vi "STATUS_Main.vi"() -> (11 "ConfigFile":path=path "/home/ArcVIEW/Modules/TCSP60/config/TCSP60_Default.cfg")   [LabVIEW 2016]
doc: "Main VI for the COMSTCP Module. This module is in charge of the externl TCP/IP comunications"
uses:
  DBSHAND/private/vis/DatabaseHand_Element_Set(string).vi
  DBSHAND/private/vis/DatabaseHand_Element_Get(string).vi
panel:
  in  "enabled":bool
  in  "updateprog":bool
  out "stop":bool
  in  "cmdstruct":cluster{"cmd":string, "respQ":string}
  out "last async.":string
  out "async":refnum<k5>
  out "error out 2":errorcluster
  in  "maxrate":sgl=0.5
  in  "maxasyncinst":i8=2
  in  "Log":bool
  in  "logfile":path
  in  "serverport":u16
  out "error out":errorcluster
  in  "Initialization Variables":string[][](table)=[["Comms", "serverport", "STATUS_Main.vi", "serverport", "1501", "U16"], ["Comms", "maxinst", "STATUS_Main.vi", "maxinst", "", "U8"], ["Misc", "maxrate", "STATUS_Main.vi", "maxrate", "", "FLOAT"], ["Misc", "updateprog", "STATUS_Main.vi", "updateprog", "", "BOOL"], ["Misc", "enabled", "STATUS_Main.vi", "enabled", "", "BOOL"], ["LOG", "file", "STATUS_Main.vi", "logfile", "", "PATH"], ["LOG", "log", "STATUS_Main.vi", "Log", "", "BOOL"]]
  in  "error in":errorcluster
  in  "ModuleName":string="STATUS"
  out "stopped":bool=TRUE
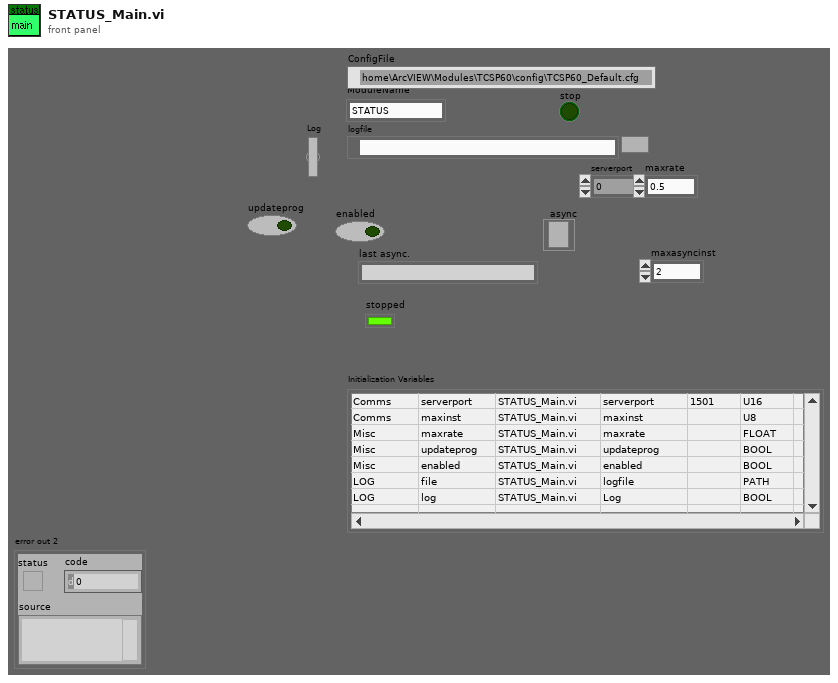
[diagram p1: front panel]
types:
  T1 = enum16{"get", "send", "delete", "add", "clean", "send_all", "send_on", "send_off"}
  T2 = typedef "DatabaseHand_RefNum.ctl" = refnum<vi>
  T3 = typedef "Status_VarsStruct.ctl" = cluster{"name":string, "value":string, "last":u32, "max":u32}
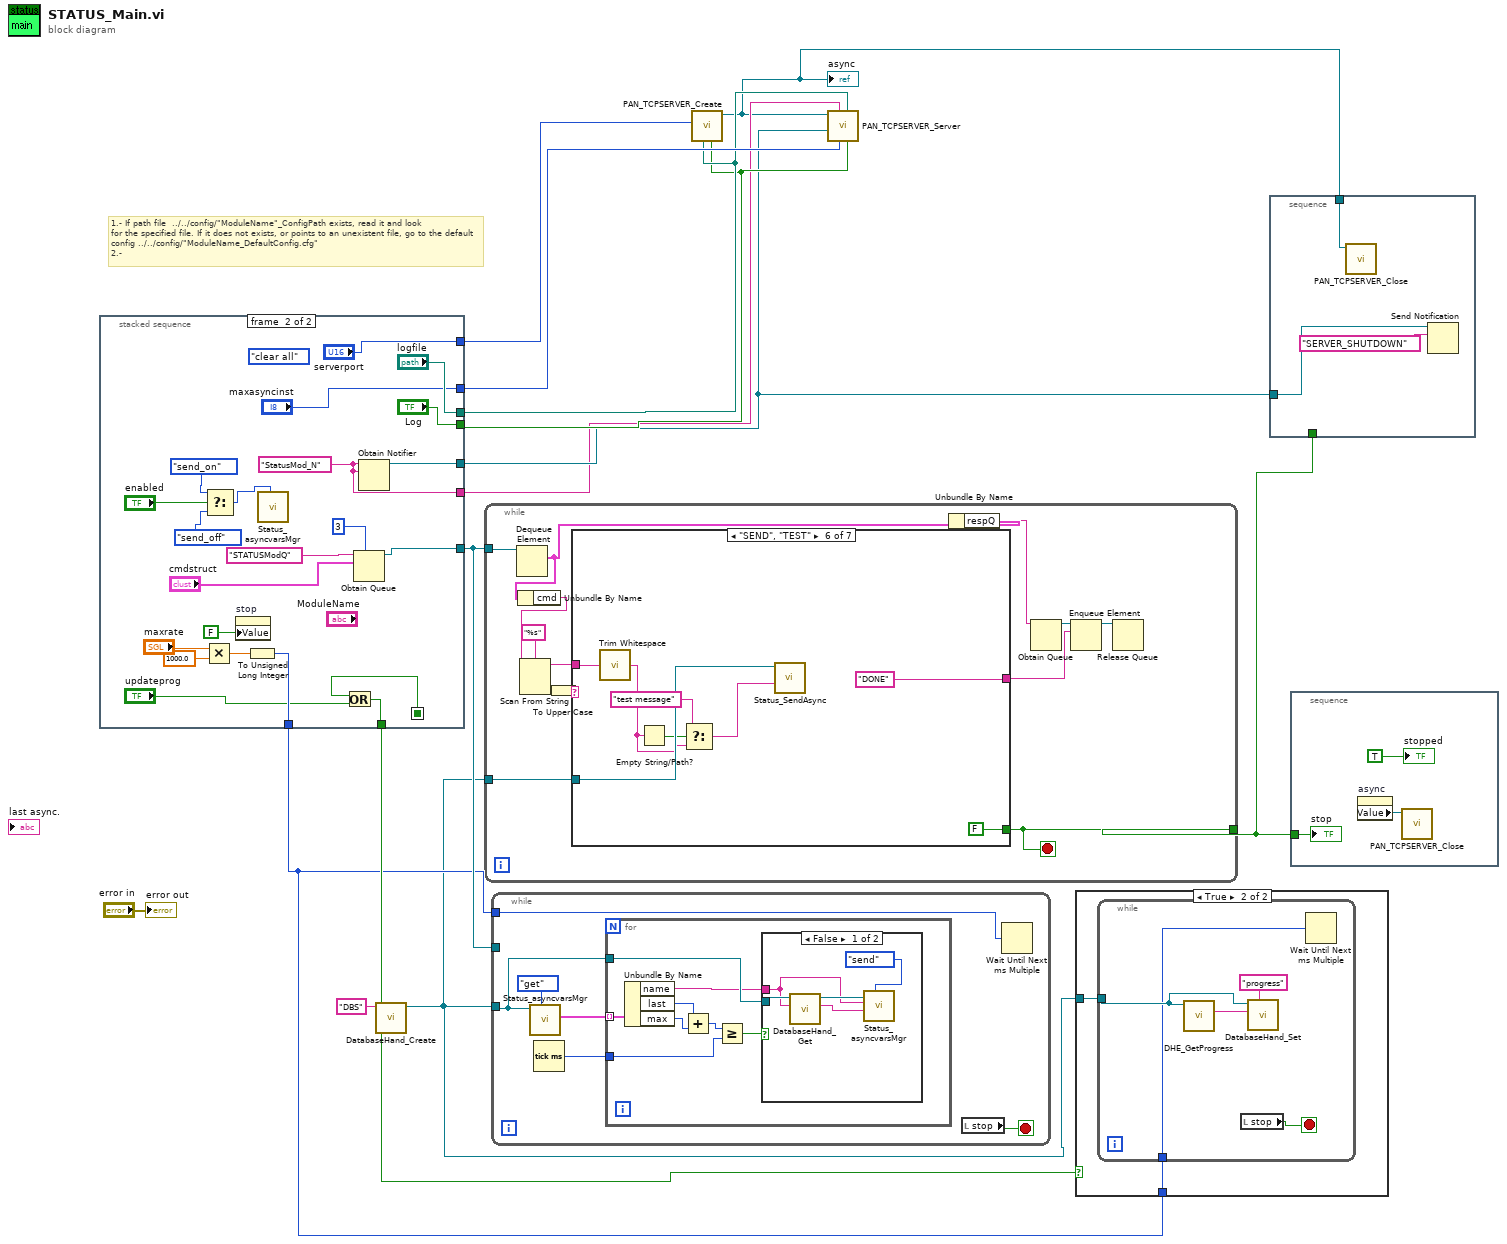
[diagram p0: block diagram]
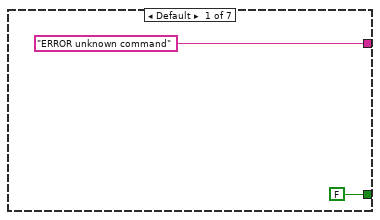
[diagram p4: hidden frame]
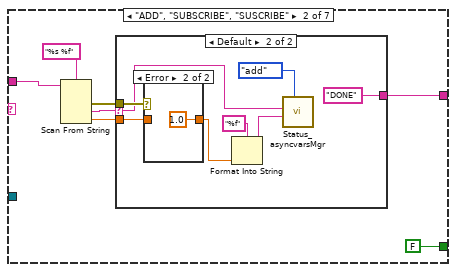
[diagram p5: hidden frame]
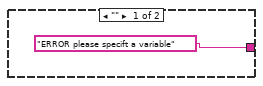
[diagram p6: hidden frame]
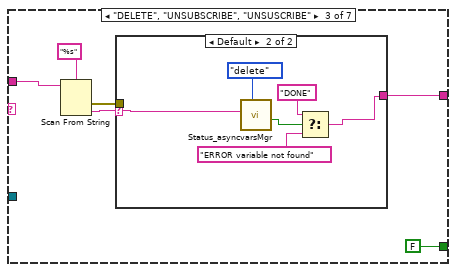
[diagram p8: hidden frame]
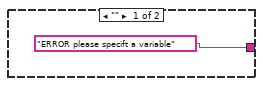
[diagram p9: hidden frame]
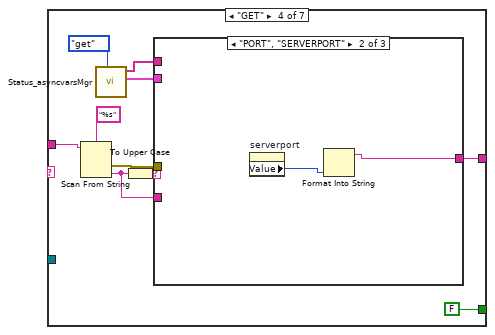
[diagram p10: hidden frame]
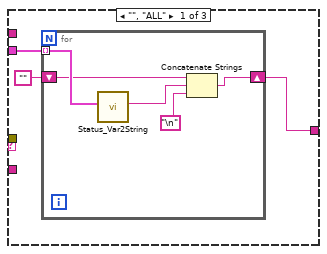
[diagram p11: hidden frame]
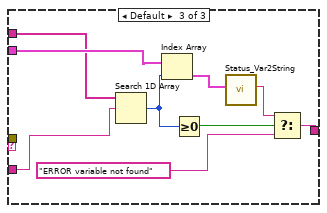
[diagram p12: hidden frame]
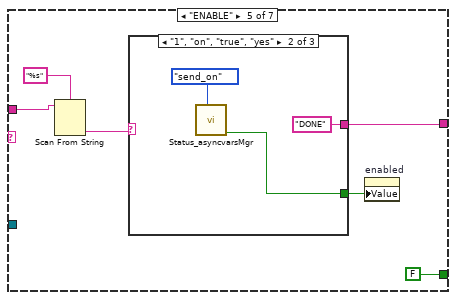
[diagram p13: hidden frame]
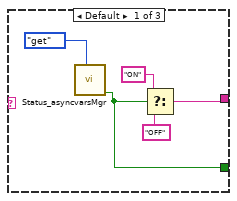
[diagram p14: hidden frame]
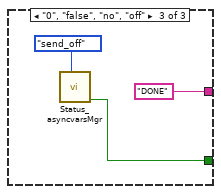
[diagram p15: hidden frame]
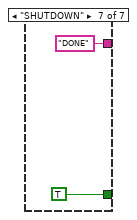
[diagram p16: hidden frame]
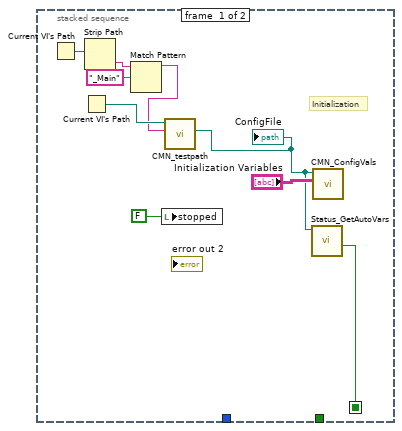
[diagram p17: hidden frame]
diagram:
  # "1.- If path file  ../../config/\"ModuleName\"_ConfigPath exists, read it and look\nfor the specified file. If it does not exists, or points to an unexistent file, go to the default\nconfig ../../config/\"ModuleName_DefaultConfig.cfg\"\n2.-"
  n1 = stacked-sequence {
    seq-local: [w15 _] -> [_ w25]
    tunnel: [_ "maxasyncinst"] -> w14
    tunnel: [_ "logfile"] -> w12
    tunnel: [_ "Log"] -> w11
    tunnel: [_ w43] -> w10
    tunnel: [_ w42] -> w9
    tunnel: [_ "serverport"] -> w8
    tunnel: [_ w36] -> w7
    tunnel: [_ w31] -> w2
    tunnel: [_ w24] -> w5
    frame #0 {
      # "Initialization"
      n2 = Current VI's Path() -> (path=w18:path)
      n3 = Current VI's Path() -> (path=w21:path)
      n4 = Strip Path(path=w18) -> (name=w19:string)  [unwired: 1 out]
      n5 = Match Pattern(string=w19, regular expression="_Main") -> (before substring=w17:string)  [unwired: 4 out]
      n6 = local write "stopped"(FALSE ("stopped")) -> ()
      n7 = call "CMN_testpath.vi"("ModuleName"=w17, "caller Path"=w21) -> ("ConfigFile"=w16:path)  [unwired: 1 in, 8 out]
      "ConfigFile" <- w16
      n8 = call "Status_GetAutoVars.vi"("ConfigFile"=w16) -> ("progress"=w15:bool)  [unwired: 1 in, 9 out]
      n9 = call "CMN_ConfigVals.vi"("ConfigVariables"="Initialization Variables", "configuration file path"=w16) -> ()  [unwired: 2 in, 8 out]
    }
    frame #1 {
      w42 = "StatusMod_N" ("name (unnamed)")
      (unwired) enum16{"add", "delete", "find", "clear all"}."clear all" ("action")
      n10 = Multiply(x="maxrate", y=sgl 1000.0) -> (x*y=w32:sgl)
      n11 = Select(t=T1."send_on" ("action"), s="enabled", f=T1."send_off" ("action")) -> (s? t:f=w28:T1)
      n12 = property on="stop" class="Bool (strict)"("Value"=FALSE ("stop")) -> ()  [unwired: 2 in, 2 out]
      n13 = To Unsigned Long Integer(number=w32) -> (unsigned 32bit integer=w31:u32)
      n14 = call "Status_asyncvarsMgr.vi"("action"=w28) -> ()  [unwired: 4 in, 7 out]
      n15 = Or(x=w25, y="updateprog") -> (x .or. y?=w24:bool)
      n16 = Obtain Queue(max queue size (-1, unlimited)=3, name (unnamed)="STATUSModQ", element data type="cmdstruct") -> (queue out=w36:refnum<queue>)  [unwired: 2 in, 2 out]
      n17 = Obtain Notifier(name (unnamed)=w42, notification data type=w42) -> (notifier out=w43:refnum<notifier>)  [unwired: 2 in, 2 out]
    }
  }
  n18 = call "DatabaseHand_Create.vi"("Name"="DBS") -> ("Database RefNum out"=w1:T2)  [unwired: 1 in, 9 out]
  n19 = while {
    tunnel: w7 -> [w58]
    tunnel: [w54] -> w3
    tunnel: w1 -> [w46]
    stop <- w54 stop-if-true
    n20 = Dequeue Element(queue=w58) -> (element=w53:cluster{"cmd":string, "respQ":string})  [unwired: 1 in, 4 out]
    n21 = Unbundle By Name(w53) -> ("cmd"=w57:string)
    n22 = Scan From String(format string="%s", input string=w57) -> (remaining string=w48:string, output 1=w55:string)  [unwired: 2 in, 3 out]
    n23 = To Upper Case(1:w55) -> (0:w47:string)
    n24 = case shown="\"SEND\", \"TEST\"" w47 {
      tunnel: [FALSE FALSE FALSE FALSE FALSE FALSE TRUE] -> w54
      tunnel: ["ERROR unknown command" ("element") w63 w80 w98 w122 "DONE" ("element") "DONE" ("element")] -> w49
      tunnel: w48 -> [_ w66 w83 w100 w125 w142 _]
      tunnel: w46 -> [_ _ _ _ _ w143 _]
      frame Default {
      }
      frame "ADD", "SUBSCRIBE", "SUSCRIBE" {
        n25 = Scan From String(format string="%s %f", input string=w66) -> (error out=w61:errorcluster, output 1=w64:string, output 2=w62:dbl)  [unwired: 2 in, 4 out]
        n26 = case shown="Default" w64 {
          selector: w64 -> [_ w73]
          tunnel: ["ERROR please specift a variable" ("element") "DONE" ("element")] -> w63
          tunnel: w62 -> [_ w75]
          tunnel: w61 -> [_ w76]
          frame "" {
          }
          frame Default {
            n27 = case shown="Error" w76 {
              tunnel: w75 -> [w77 _]
              tunnel: [w77 1.0] -> w72
              frame No Error {
              }
              frame Error {
              }
            }
            n28 = Format Into String(format string="%f", w72) -> (resulting string=w71:string)  [unwired: 2 in, 1 out]
            n29 = call "Status_asyncvarsMgr.vi"("action"=T1."add", "value"=w71, "var"=w73) -> ()  [unwired: 2 in, 7 out]
          }
        }
      }
      frame "DELETE", "UNSUBSCRIBE", "UNSUSCRIBE" {
        n30 = Scan From String(format string="%s", input string=w83) -> (error out=w79:errorcluster, output 1=w81:string)  [unwired: 2 in, 3 out]
        n31 = case shown="Default" w81 {
          selector: w81 -> [_ w90]
          tunnel: ["ERROR please specift a variable" ("element") w87] -> w80
          tunnel: w79 -> [_ _]
          frame "" {
          }
          frame Default {
            n32 = call "Status_asyncvarsMgr.vi"("action"=T1."delete", "var"=w90) -> ("found"=w89:bool)  [unwired: 3 in, 6 out]
            n33 = Select(t="DONE" ("element"), s=w89, f="ERROR variable not found") -> (s? t:f=w87:string)
          }
        }
      }
      frame "GET" {
        n34 = Scan From String(format string="%s", input string=w100) -> (error out=w97:errorcluster, output 1=w93:string)  [unwired: 2 in, 3 out]
        n35 = call "Status_asyncvarsMgr.vi"("action"=T1."get") -> ("vars"=w95:T3[], "names"=w94:string[])  [unwired: 4 in, 5 out]
        n36 = To Upper Case(1:w93) -> (0:w92:string)
        n37 = case shown="\"PORT\", \"SERVERPORT\"" w92 {
          tunnel: [w103 w110 w118] -> w98
          tunnel: w97 -> [_ _ _]
          tunnel: w95 -> [w104 _ w114]
          tunnel: w94 -> [_ _ w113]
          tunnel: w93 -> [_ _ w112]
          frame "", "ALL" {
            n38 = for {
              tunnel: w104 -> [w109] mode=indexing
              shift-right: [w106] -> w103
              shift-left: "" -> [w105]
              n39 = call "Status_Var2String.vi"("element"=w109) -> ("resulting string"=w108:string)  [unwired: 10 out]
              n40 = Concatenate Strings(w105, w108, "\n") -> (w106:string)
            }
          }
          frame "PORT", "SERVERPORT" {
            n41 = property on="serverport" class="DigNum (strict)"() -> ("Value"=w111:u16)  [unwired: 2 in, 2 out]
            n42 = Format Into String(w111) -> (resulting string=w110:string)  [unwired: 3 in, 1 out]
          }
          frame Default {
            n43 = Search 1D Array(1D array=w113, element=w112) -> (index of element=w117:i32)  [unwired: 1 out]
            n44 = Index Array(array=w114, index=w117) -> (element=w116:T3)
            n45 = Greater Or Equal To 0?(x=w117) -> (x >= 0?=w120:bool)
            n46 = call "Status_Var2String.vi"("element"=w116) -> ("resulting string"=w115:string)  [unwired: 10 out]
            n47 = Select(t=w115, s=w120, f="ERROR variable not found") -> (s? t:f=w118:string)
          }
        }
      }
      frame "ENABLE" {
        n48 = Scan From String(format string="%s", input string=w125) -> (output 1=w123:string)  [unwired: 2 in, 4 out]
        n49 = case shown="\"1\", \"on\", \"true\", \"yes\"" w123 {
          tunnel: [w129 "DONE" ("element") "DONE" ("element")] -> w122
          tunnel: [w127 w132 w135] -> w121
          frame Default {
            n50 = call "Status_asyncvarsMgr.vi"("action"=T1."get") -> ("enabled"=w127:bool)  [unwired: 4 in, 6 out]
            n51 = Select(t="ON" ("element"), s=w127, f="OFF") -> (s? t:f=w129:string)
          }
          frame "1", "on", "true", "yes" {
            n52 = call "Status_asyncvarsMgr.vi"("action"=T1."send_on") -> ("enabled"=w132:bool)  [unwired: 4 in, 6 out]
          }
          frame "0", "false", "no", "off" {
            n53 = call "Status_asyncvarsMgr.vi"("action"=T1."send_off") -> ("enabled"=w135:bool)  [unwired: 4 in, 6 out]
          }
        }
        n54 = property on="enabled" class="Bool (strict)"("Value"=w121) -> ()  [unwired: 2 in, 2 out]
      }
      frame "SEND", "TEST" {
        n55 = call <vilib>:"Trim Whitespace.vi"("string"=w142) -> ("trimmed string"=w139:string)  [unwired: 1 in]
        n56 = Empty String/Path?(string/path=w139) -> (empty?=w141:bool)
        n57 = Select(t="test message" ("Message"), s=w141, f=w139) -> (s? t:f=w138:string)
        n58 = call "Status_SendAsync.vi"("Message"=w138, "Database RefNum in"=w143) -> ()  [unwired: 1 in, 9 out]
      }
      frame "SHUTDOWN" {
      }
    }
    n59 = Unbundle By Name(w53) -> ("respQ"=w52:string)
    n60 = Obtain Queue(name (unnamed)=w52, element data type=w52) -> (queue out=w51:refnum<queue>)  [unwired: 3 in, 2 out]
    n61 = Enqueue Element(queue=w51, element=w49) -> (queue out=w50:refnum<queue>)  [unwired: 1 in, 3 out]
    n62 = Release Queue(queue=w50) -> ()  [unwired: 1 in, 4 out]
  }
  n63 = while {
    tunnel: w7 -> [_]
    tunnel: w1 -> [w149]
    tunnel: w2 -> [w148]
    stop <- w153 stop-if-true
    n64 = call "Status_asyncvarsMgr.vi"("action"=T1."get", "Database RefNum in"=w149) -> ("vars"=w151:T3[])  [unwired: 3 in, 6 out]
    n65 = Tick Count (ms)() -> (millisecond timer value=w150:u32)
    n66 = for {
      tunnel: w151 -> [w161] mode=indexing
      tunnel: w150 -> [w158]
      tunnel: w149 -> [w156]
      n67 = Unbundle By Name(w161) -> ("name"=w155:string, "last"=w160:u32, "max"=w154:u32)
      n68 = Add(x=w160, y=w154) -> (x+y=w159:u32)
      n69 = Greater Or Equal?(x=w159, y=w158) -> (x >= y?=w157:bool)
      n70 = case shown="False" w157 {
        tunnel: w156 -> [w166 _]
        tunnel: w155 -> [w163 _]
        frame False {
          n71 = call-poly "DatabaseHand_Get.vi"("name"=w163, "Database RefNum in"=w166) -> ("value"=w162:string, "Database RefNum out"=w164:T2)  [unwired: 3 in, 5 out]
          n72 = call "Status_asyncvarsMgr.vi"("action"=T1."send", "value"=w162, "var"=w163, "Database RefNum in"=w164) -> ()  [unwired: 1 in, 7 out]
        }
        frame True {
        }
      }
    }
    n73 = local read "stop"() -> (w153:bool)
    n74 = Wait Until Next ms Multiple(millisecond multiple=w148) -> ()  [unwired: 1 out]
  }
  n75 = call "PAN_TCPSERVER_Create.vi"("log"=w11, "logfile"=w12, "port"=w8) -> ("listener ID"=w4:refnum<k5>)  [unwired: 2 in, 6 out]
  "async" <- w4
  n76 = call "PAN_TCPSERVER_Server.vi"("log"=w11, "logfile"=w12, "max instances"=w14, "callerID"=w9, "notifier In"=w10, "listener ID"=w4) -> ()  [unwired: 2 in, 4 out]
  n77 = case shown="True" w5 {
    tunnel: w1 -> [_ w168]
    tunnel: w2 -> [_ w167]
    frame False {
    }
    frame True {
      n78 = while {
        tunnel: w168 -> [w172]
        tunnel: w167 -> [w169]
        stop <- w173 stop-if-true
        n79 = call "DHE_GetProgress.vi"("Databse Ref"=w172) -> ("progress"=w171:string)  [unwired: 1 in, 9 out]
        n80 = local read "stop"() -> (w173:bool)
        n81 = call-poly "DatabaseHand_Set.vi"("name"="progress", "value"=w171, "Database RefNum in"=w172) -> ()  [unwired: 5 in, 4 out]
        n82 = Wait Until Next ms Multiple(millisecond multiple=w169) -> ()  [unwired: 1 out]
      }
    }
  }
  n83 = stacked-sequence {
    tunnel: w10 -> [w175]
    tunnel: w4 -> [w174]
    tunnel: w3 -> [_]
    frame #0 {
      n84 = call "PAN_TCPSERVER_Close.vi"("listener ID"=w174) -> ()  [unwired: 1 in, 10 out]
      n85 = Send Notification(notification="SERVER_SHUTDOWN", notifier=w175) -> ()  [unwired: 1 in, 2 out]
    }
  }
  n86 = stacked-sequence {
    tunnel: w3 -> [w177]
    frame #0 {
      n87 = property on="async" class="Ref (strict)"() -> ("Value"=w178:refnum<k5>)  [unwired: 2 in, 2 out]
      n88 = call "PAN_TCPSERVER_Close.vi"("listener ID"=w178) -> ()  [unwired: 1 in, 10 out]
      "stopped" <- TRUE
      "stop" <- w177
    }
  }
  "error out" <- "error in"
